vi "Nano-drive set xyz.vi"(0 "X (um)":sgl min=0 max=100 format="%.4f", 1 "Board ID":u16=1 min=1, 2 "Y (um)":sgl min=0 max=100 format="%.4f", 3 "Z (um)":sgl min=0 max=100 format="%.4f", 4 "Set this axis?":cluster{"X":bool, "Y":bool, "Z":bool}) -> ()   [LabVIEW 2011]
uses:
  MCLib.dll
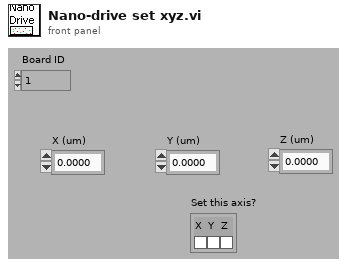
[diagram p1: front panel]
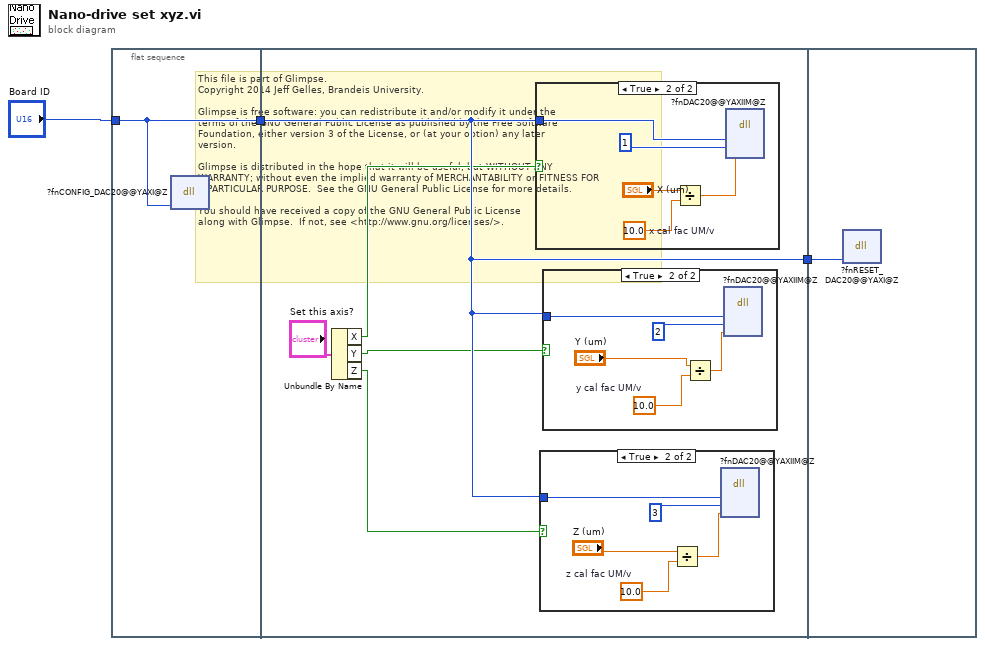
[diagram p0: block diagram]
diagram:
  # "This file is part of Glimpse. \nCopyright 2014 Jeff Gelles, Brandeis University.    \n\nGlimpse is free software: you can redistribute it and/or modify it under the \nterms of the GNU General Public License as published by the Free Software \nFoundation, either version 3 of the License, or (at your option) any later \nversion.\n\nGlimpse is distributed in the hope that it will be useful, but WITHOUT ANY \nWARRANTY; without even the implied warranty of MERCHANTABILITY or FITNESS FOR \nA PARTICULAR PURPOSE.  See the GNU General Public License for more details.\n\nYou should have received a copy of the GNU General Public License\nalong with Glimpse.  If not, see <http://www.gnu.org/licenses/>."
  n1 = flat-sequence {
    tunnel: "Board ID" -> [w4]
    tunnel: [w4] -> w2
    tunnel: w2 -> [w9]
    tunnel: [w9] -> w1
    tunnel: w1 -> [w25]
    frame #0 {
      n2 = dll-call lib="//MCLib.dll" fn="?fnCONFIG_DAC20@@YAXI@Z" label="fnCONFIG_DAC20"(w4) -> ()  [unwired: 5 in, 2 out]
    }
    frame #1 {
      n3 = Unbundle By Name("Set this axis?") -> ("X"=w7:bool, "Y"=w6:bool, "Z"=w5:bool)
      n4 = case shown="True" w7 {
        tunnel: w9 -> [_ w24]
        frame False {
        }
        frame True {
          w22 = 10.0  # x cal fac UM/v
          n5 = Divide(x="X (um)", y=w22) -> (x/y=w20:dbl)
          n6 = dll-call lib="//MCLib.dll" fn="?fnDAC20@@YAXIIM@Z" label="fnDAC20"(w24, 1, w20) -> ()  [unwired: 7 in, 2 out]
        }
      }
      n7 = case shown="True" w5 {
        tunnel: w9 -> [_ w13]
        frame False {
        }
        frame True {
          w12 = 10.0  # z cal fac UM/v
          n8 = Divide(x="Z (um)", y=w12) -> (x/y=w10:dbl)
          n9 = dll-call lib="//MCLib.dll" fn="?fnDAC20@@YAXIIM@Z"(w13, 3, w10) -> ()  [unwired: 7 in, 2 out]
        }
      }
      n10 = case shown="True" w6 {
        tunnel: w9 -> [_ w18]
        frame False {
        }
        frame True {
          w17 = 10.0  # y cal fac UM/v
          n11 = Divide(x="Y (um)", y=w17) -> (x/y=w15:dbl)
          n12 = dll-call lib="//MCLib.dll" fn="?fnDAC20@@YAXIIM@Z"(w18, 2, w15) -> ()  [unwired: 7 in, 2 out]
        }
      }
    }
    frame #2 {
      n13 = dll-call lib="//MCLib.dll" fn="?fnRESET_DAC20@@YAXI@Z" label="fnRESET_DAC20"(w25) -> ()  [unwired: 5 in, 2 out]
    }
  }
